vi "Sort Main Properties.vi"(8 "error in (no error)":errorcluster, 11 "Item Ref in":T1 format="%.0x") -> (0 "error out":errorcluster, 2 "Channel Config":T2)   [LabVIEW 2021, in "Software Multi-Plex System Explorer.lvlib"]
uses:
  Software Multi-Plex System Explorer.lvlib
  Types/Channel Config.ctl
  Types/Index Type.ctl
  <vilib>/NI VeriStand/Custom Device API/Custom Device Item Ref.ctl
  Shared/Constants.vi
  <vilib>/NI VeriStand/Custom Device Tools/Custom Device Utility Library/NI VeriStand - Search for All Items by GUID.vi
  <vilib>/NI VeriStand/Custom Device Tools/Custom Device Utility Library/Custom Device Utility Library.lvlib
  Shared/Software Multi-Plex Shared.lvlib
  <vilib>/NI VeriStand/Custom Device API/Custom Device API.lvlib
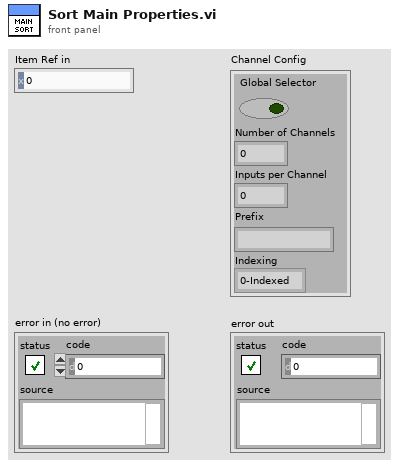
[diagram p1: front panel]
types:
  T1 = typedef "Custom Device API.lvlib/Custom Device Item Ref.ctl" = u64
  T2 = typedef "Software Multi-Plex System Explorer.lvlib/Channel Config.ctl" = cluster{"Global Selector":bool, "Number of Channels":i32, "Inputs per Channel":i32, "Prefix":string, "Indexing":T3}
  T3 = typedef "Software Multi-Plex System Explorer.lvlib/Index Type.ctl" = enum16{"0-Indexed", "1-Indexed"}
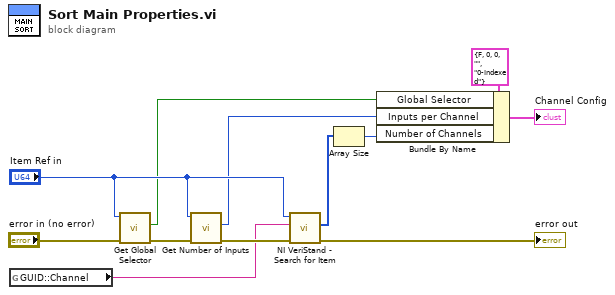
[diagram p0: block diagram]
diagram:
  n1 = global read "Constants.vi" "GUID::Channel"() -> (w8:string)
  n2 = call "Get Global Selector.vi"("error in (no error)"="error in (no error)", "Item Ref in"="Item Ref in") -> ("error out"=w11:errorcluster, "Global Selector"=w6:bool)  [unwired: 8 in]
  n3 = call "Get Number of Inputs.vi"("error in (no error)"=w11, "Item Ref in"="Item Ref in") -> ("error out"=w10:errorcluster, "Number of Inputs"=w5:i32)  [unwired: 8 in]
  n4 = call-poly <vilib>:"NI VeriStand - Search for Item.vi"("error in"=w10, "Item GUID"=w8, "Section Ref in"="Item Ref in") -> ("error out"=→"error out":errorcluster, "Item Refs"=w3:T1[])  [unwired: 5 in, 2 out]
  n5 = Array Size(array=w3) -> (size(s)=w4:i32)
  n6 = Bundle By Name(cluster=T2 {"Global Selector"=FALSE, "Number of Channels"=0, "Inputs per Channel"=0, "Prefix"="", "Indexing"=enum."0-Indexed"} ("Channel Config"), "Global Selector"=w6, "Inputs per Channel"=w5, "Number of Channels"=w4) -> (→"Channel Config":T2)
